vi "read_test_log_file.vi"(8 "error in (no error)":errorcluster, 11 "file path (use dialog)":path) -> (0 "error out":errorcluster, 3 "JSON content":string)   [LabVIEW 2015]
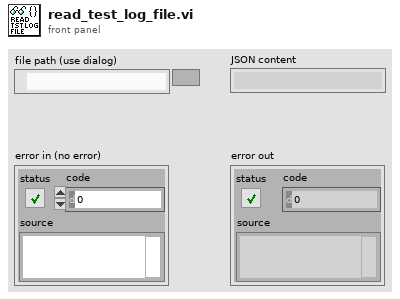
[diagram p1: front panel]
types:
  T1 = enum16{"open", "replace", "create", "open or create", "replace or create", "replace or create with confirmation"}
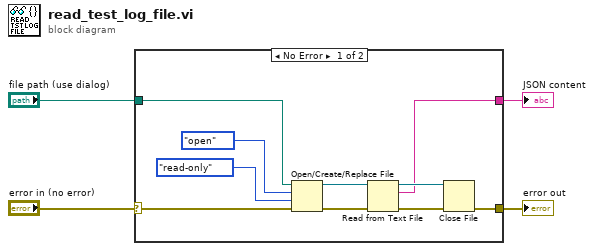
[diagram p0: block diagram]
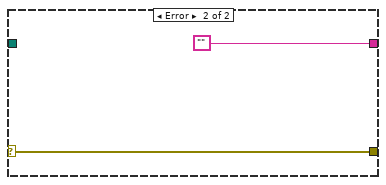
[diagram p2: hidden frame]
diagram:
  n1 = case shown="No Error" "error in (no error)" {
    selector: "error in (no error)" -> [w7 w16]
    tunnel: [w8 w16] -> w4
    tunnel: "file path (use dialog)" -> [w6 _]
    tunnel: [w5 ""] -> w1
    frame No Error {
      n2 = Open/Create/Replace File(file path (use dialog)=w6, error in=w7, operation (0:open)=T1."open", access (0:read/write)=enum16{"read/write", "read-only", "write-only"}."read-only") -> (refnum out=w12:refnum<file>, error out=w13:errorcluster)  [unwired: 2 in, 1 out]
      n3 = Read from Text File(file (use dialog)=w12, error in=w13) -> (refnum out=w10:refnum<file>, text=w5:string, error out=w11:errorcluster)  [unwired: 2 in, 1 out]
      n4 = Close File(refnum=w10, error in=w11) -> (error out=w8:errorcluster)  [unwired: 1 out]
    }
    frame Error {
    }
  }
  "error out" <- w4
  "JSON content" <- w1
